vi "数据摘要显示.vi"(10 "删除？":bool[](array[boolean]), 11 "数据摘要":string[][](array[string])) -> ()   [LabVIEW 2020]
uses:
  097fb45d-801a-408a-8776-59581c35b5b4.vi
  095f5dbe-0725-4b36-8b67-90435d1a6c1a.vi
  097fb45d-801a-408a-8776-59581c35b5b4.vi/0dc45aae-b235-4892-9b42-dacecac7f01c.vi
  095f5dbe-0725-4b36-8b67-90435d1a6c1a.vi/0dc45aae-b235-4892-9b42-dacecac7f01c.vi
panel:
  out "显示":string[][](table)
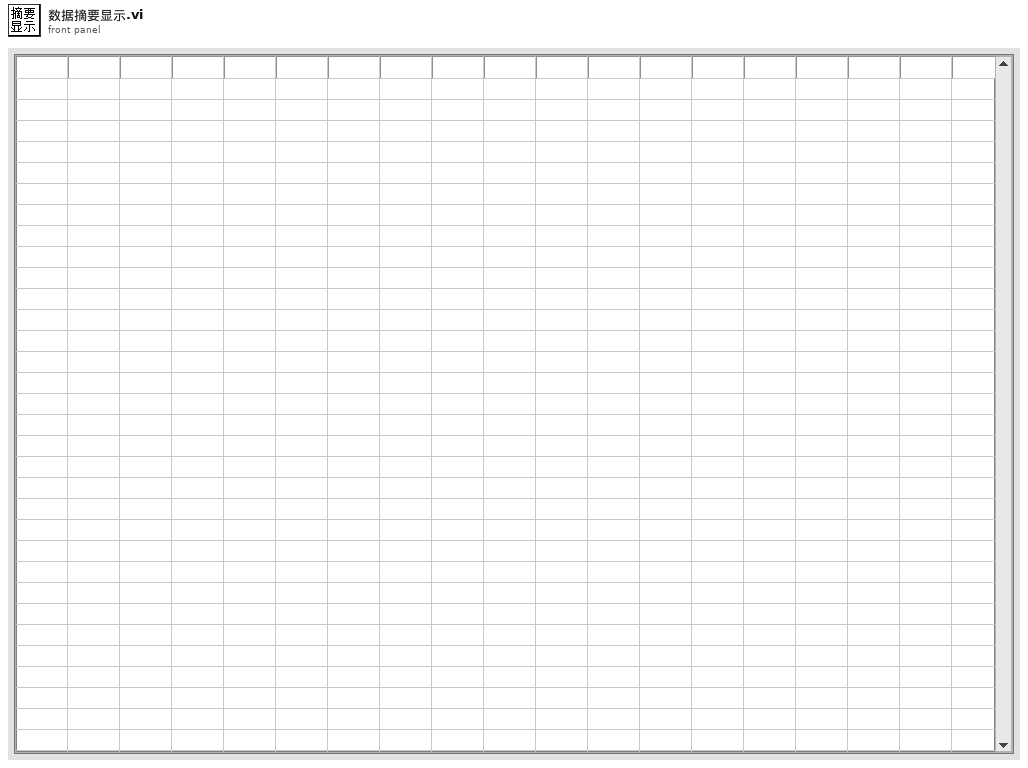
[diagram p1: front panel]
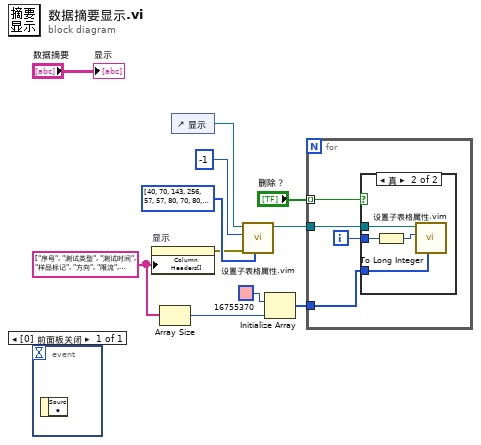
[diagram p0: block diagram]
diagram:
  w2 = string[] ["序号", "测试类型", "测试时间", "样品标记", "方向", "限流", "总时长", "数据量", "测试电压", "突变电压", "循环"] ("列首字符串[]")
  n1 = event shown="[0] 前面板关闭" {
    selector: _ -> [_]
    dyn-events: _ -> [_]
    timeout: _ -> [_]
    event Panel Close {
      n2 = event-data() -> ()  [unwired: 1 in, 1 out]
    }
  }
  n3 = property on="显示" class="Tbl (严格)"("Column Headers[]"=w2) -> (error out=w1:errorcluster)  [unwired: 2 in, 1 out]
  n4 = Array Size(array=w2) -> (size(s)=w5:i32)
  n5 = control-ref of="显示"() -> (w9:refnum<vi>)
  n6 = call "设置子表格属性.vim"("子表格属性"=u16[] [40, 70, 143, 256, 57, 57, 80, 70, 80, 80, 35] ("数组"), "错误输入（无错误）"=w1, "Row"=-1, "表格引用输入"=w9) -> ("表格引用输出"=w7:refnum<vi>)  [unwired: 6 in, 1 out]
  n7 = Initialize Array(u32 16755370, w5) -> (w4:u32[])
  n8 = for {
    tunnel: w7 -> [w15]
    tunnel: "删除？" -> [w14] mode=indexing
    tunnel: w4 -> [w12]
    i -> [w13]
    n9 = case shown="真" w14 {
      tunnel: w15 -> [_ w19]
      tunnel: w13 -> [_ w18]
      tunnel: w12 -> [_ w17]
      frame False {
      }
      frame True {
        n10 = To Long Integer(number=w18) -> (32bit integer=w16:i32)
        n11 = call "设置子表格属性.vim"("子表格属性"=w17, "Row"=w16, "表格引用输入"=w19) -> ()  [unwired: 7 in, 2 out]
      }
    }
  }
  "显示" <- "数据摘要"
